vi "ResetNode.vi"(10 "overhaul count":i32, 11 "node reference in":refnum<data-value>) -> (3 "node reference out":refnum<data-value>)   [LabVIEW 2013, in "RVCLibrary_Bug2.lvclass"]
uses:
  RVCLibrary_Bug2.lvclass
  <vilib>/robotics/Navigation/shared/MapNode/AbstractDstarNode/NI_Robotics_AbstractDstarNode.lvclass
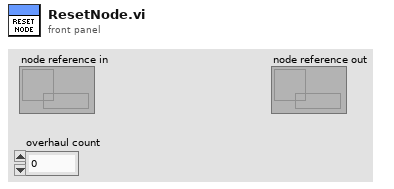
[diagram p1: front panel]
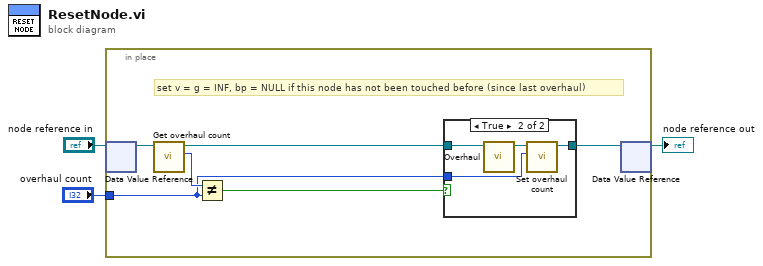
[diagram p0: block diagram]
diagram:
  n1 = in-place {
    in-place-border: "overhaul count" -> [w4]
    # "set v = g = INF, bp = NULL if this node has not been touched before (since last overhaul)"
    n2 = in-place-dvr #1("node reference in") -> (w9:refnum<class "NI_Robotics_AbstractDstarNode.lvclass">)  [unwired: 1 out]
    n3 = call <vilib>:"Get overhaul count.vi"("AbstractDstarNode in"=w9) -> ("overhaul count"=w8:i32, "AbstractDstarNode out"=w7:refnum<class "NI_Robotics_AbstractDstarNode.lvclass">)  [unwired: 9 in]
    n4 = Not Equal?(x=w8, y=w4) -> (x != y?=w6:bool)
    n5 = case shown="True" w6 {
      tunnel: w7 -> [w10 w14]
      tunnel: [w10 w12] -> w5
      tunnel: w4 -> [_ w11]
      frame False {
      }
      frame True {
        n6 = call <vilib>:"Overhaul.vi"("AbstractDstarNode in"=w14) -> ("AbstractDstarNode out"=w13:refnum<class "NI_Robotics_AbstractDstarNode.lvclass">)  [unwired: 10 in]
        n7 = call <vilib>:"Set overhaul count.vi"("overhaul count"=w11, "AbstractDstarNode in"=w13) -> ("AbstractDstarNode out"=w12:refnum<class "NI_Robotics_AbstractDstarNode.lvclass">)  [unwired: 9 in]
      }
    }
    n8 = in-place-dvr #1(w5) -> (→"node reference out":refnum<data-value>)  [unwired: 1 out]
  }
